vi "Basic_Acquire_Widefield_test.vi"() -> ()   [LabVIEW 2009]
uses:
  <vilib>/vision/Image Controls.llb/IMAQ Image.ctl
  <vilib>/userDefined/High Color/IMAQdx.ctl
  Widefield_globals.vi
  <vilib>/DAQmx/create/channels.llb/DAQmx Create Channel (DO-Digital Output).vi
  <vilib>/DAQmx/configure/timing.llb/DAQmx Timing (Implicit).vi
  <vilib>/DAQmx/create/channels.llb/DAQmx Create Channel (CO-Pulse Generation-Ticks).vi
  <vilib>/Platform/TimedLoop/XDataNode/XDataNode.xnode
  <vilib>/Platform/TimedLoop/XDataNode/loadlvalarms.vi
  <vilib>/Platform/TimedLoop/XDataNode/timing_clust.ctl
  <vilib>/Platform/TimedLoop/XDataNode/nitl_modes.ctl
  <vilib>/Platform/TimedLoop/XDataNode/wakeup.ctl
  <vilib>/DAQmx/write.llb/DAQmx Write (Digital Bool 1Line 1Point).vi
  Program Files/National Instruments/LabVIEW 2009/resource/objmgr/imaqdx.rc
  <vilib>/vision/driver/NI_Vision_Acquisition_Software.lvlib
  <vilib>/Platform/TimedLoop/XDataNode/XDNodeRunTimeDep.lvlib
panel:
  in  "y":dbl
  out "x*y":dbl
  out "RatioIm 2":u8[][](graph)
  out "frame number":i32
  out "IMAQ session":T1 caption="Session Out"
  out "frame times":i32[](array[numeric])
  out "error out":errorcluster
  out "LED settle":i32
  out "Control LED?":bool
  out "stim tag":string
  out "SF file":string
  out "One Bulb?":bool
  out "File Path":path
  out "SingleFrames":bool
  out "empty frame":dbl[][](array[numeric])
  out "Resolution":u32[](array[numeric])
  out "Experiment Sequence":dbl[][](array[numeric])
  out "settings":sgl[](array[numeric])
  out "Buff Img":T2
  out "COString":string
  in  "Offset (32768 default)":u32=32768
  in  "Contrast (600000 default)":u32=600000
  in  "Pause":bool=TRUE
  out "ExpOrderRefnum":refnum<file>
  out "Subframes":u32
  out "DCSAir":dbl[][](array[numeric])
  out "DCOdor":dbl[][](array[numeric])
  out "DCAir":dbl[][](array[numeric])
  out "TiffRefnum":refnum<file>
  out "Indices":i32[](array[numeric])
  out "Frames SAir":u32
  out "Odors:":u32
  out "StopAcq":bool
  in  "Stop":bool=TRUE
  out "Odor #":i32=50
  out "Repeats:":i32=1
  out "Repeat #":i32=1
  out "Frames Odor":u32
  out "Frames Air":u32
  out "Status":string
  out "Stimulus #":i32
  in  "start":bool=TRUE
  # "Filtered Ratio Image"
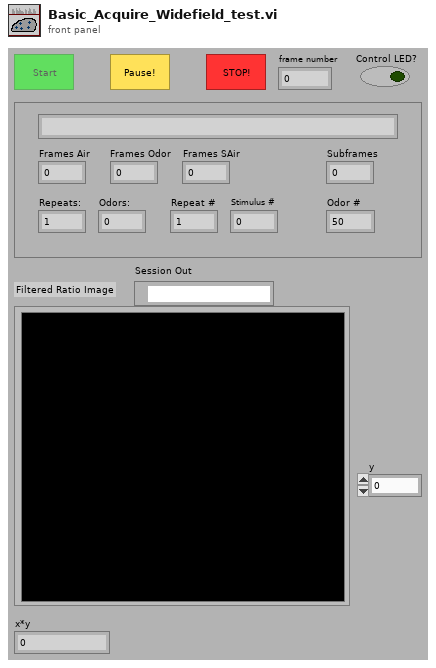
[diagram p1: front panel]
types:
  T1 = typedef "IMAQdx.ctl" = refnum<k21>
  T2 = typedef "IMAQ Image.ctl" = refnum<image>
  T3 = enum16{"open", "replace", "create", "open or create", "replace or create", "replace or create with confirmation"}
  T4 = typedef "XDNodeRunTimeDep.lvlib/timing_clust.ctl" = cluster{"Expected End [f-1]":u64, "Actual End [f-1]":u64, "Finished Late? [f-1]":bool, "Expected End [i-1]":u64, "Actual End [i-1]":u64, "Finished Late? [i-1]":bool, "Expected Start [i]":u64, "Actual Start [i]":u64, "Expected Start [f]":u64, "Actual Start [f]":u64, "Source Name":string, "Structure Name":string, "Period":i64, "Deadline":i64, "Offset":i64, "Start":i64, "Priority":i32, "Timeout":i32, "Mode":T5, "Wakeup Reason":T6, "Error":errorcluster, "Source Type":string, "Secondary Source Type":string, "Global End Time":u64, "Global Start Time":u64, "Frame Duration":u64, "Iteration Duration":u64, "Assigned CPU":i32, "I/O Scan Engine Mode":u32}
  T5 = typedef "XDNodeRunTimeDep.lvlib/nitl_modes.ctl" = enum32{"No Change", "Process missed periods, maintain original phase", "Discard missed periods, maintain original phase", "Process missed periods, ignore original phase", "Discard missed periods, ignore original phase"}
  T6 = typedef "XDNodeRunTimeDep.lvlib/wakeup.ctl" = enum32{"Normal", "Aborted", "Asynchronous wakeup", "Timing source error", "Timed loop error", "Timeout"}
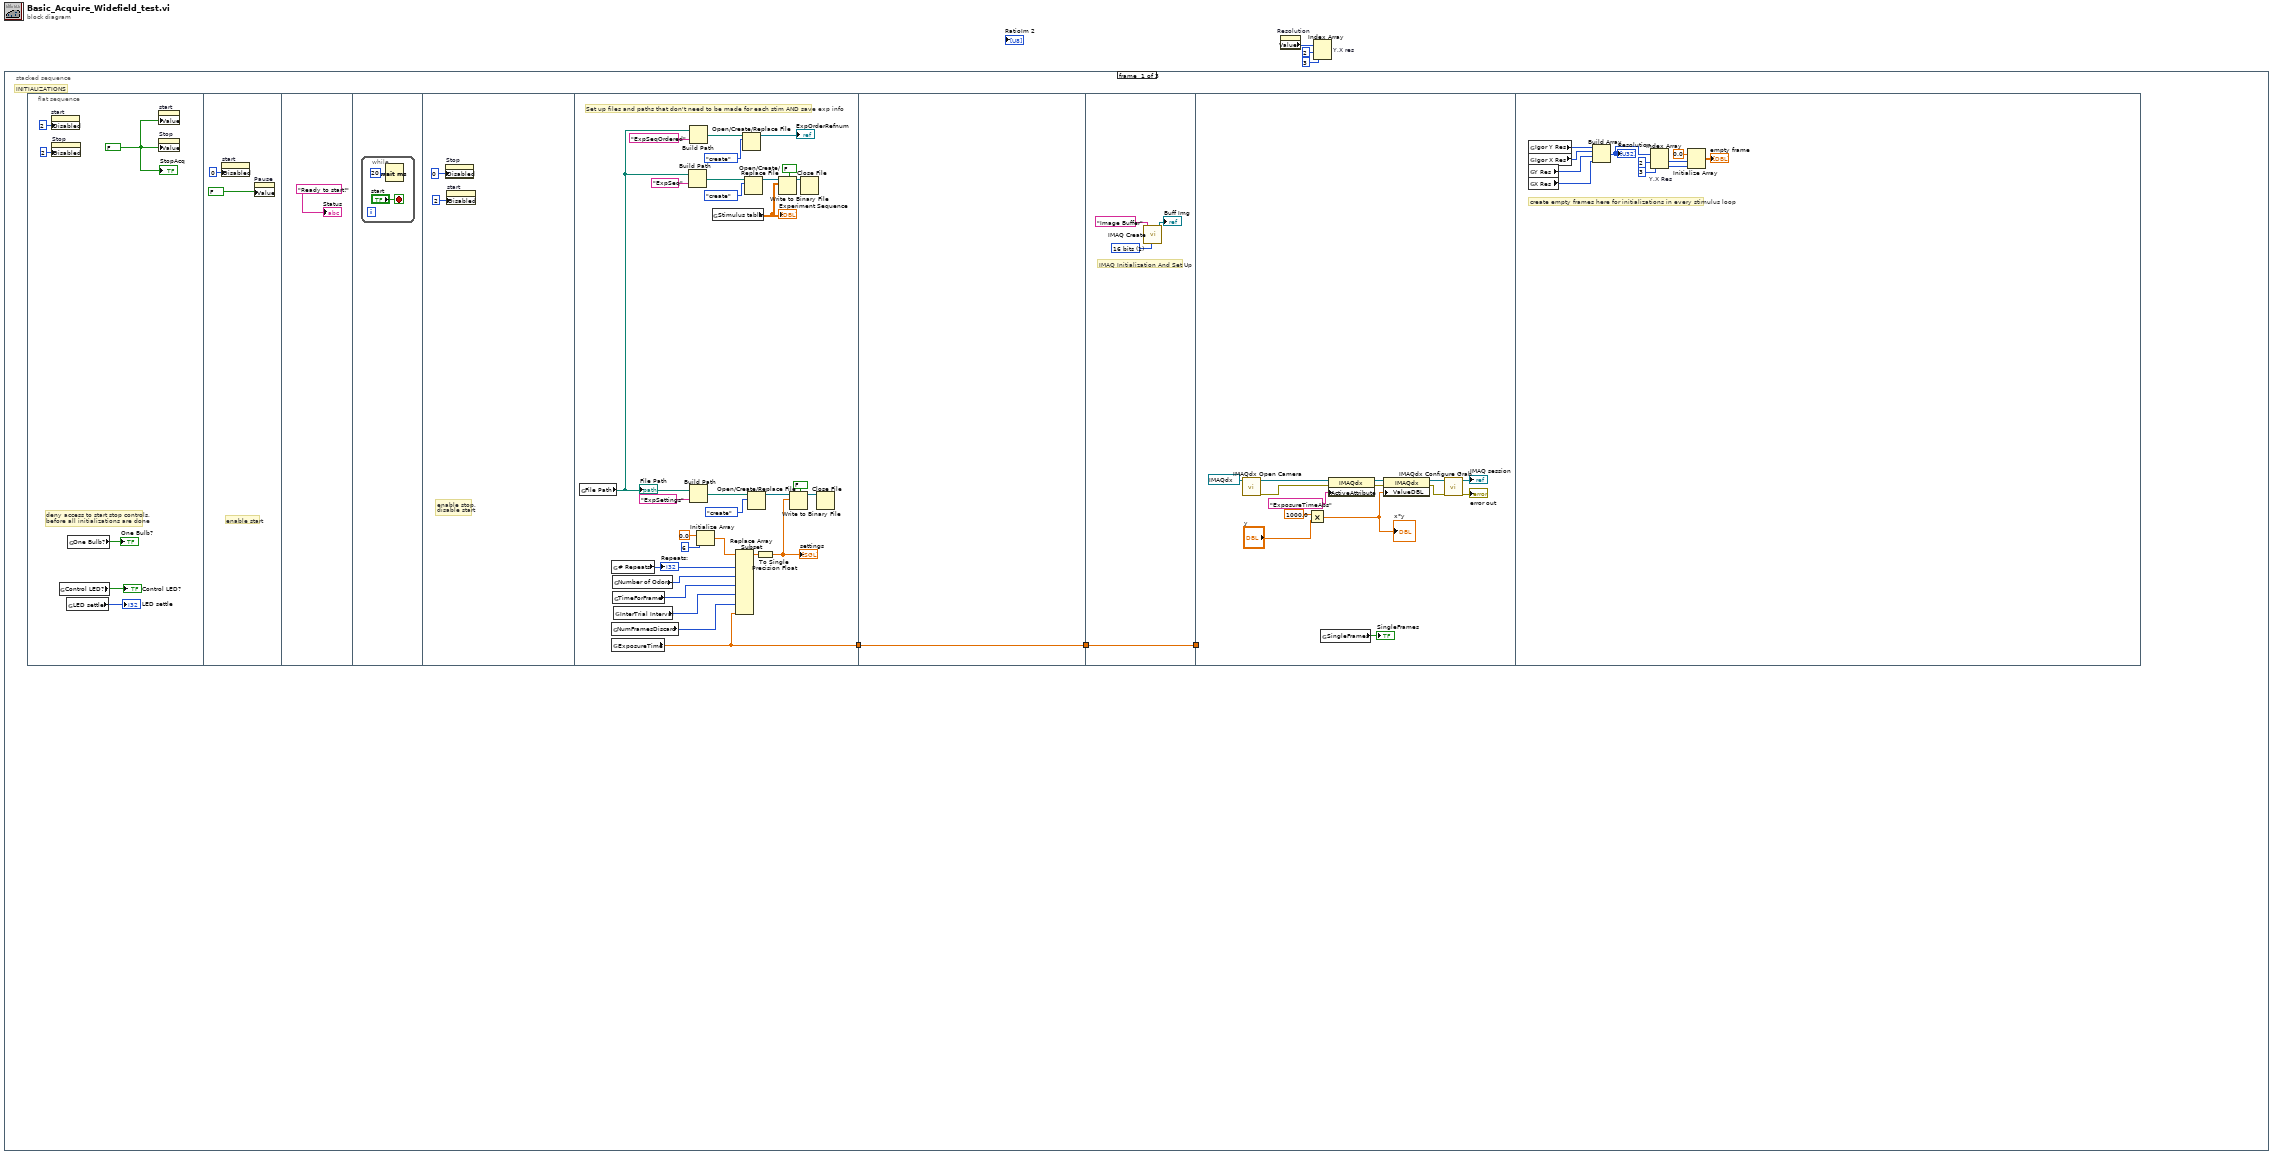
[diagram p0: block diagram]
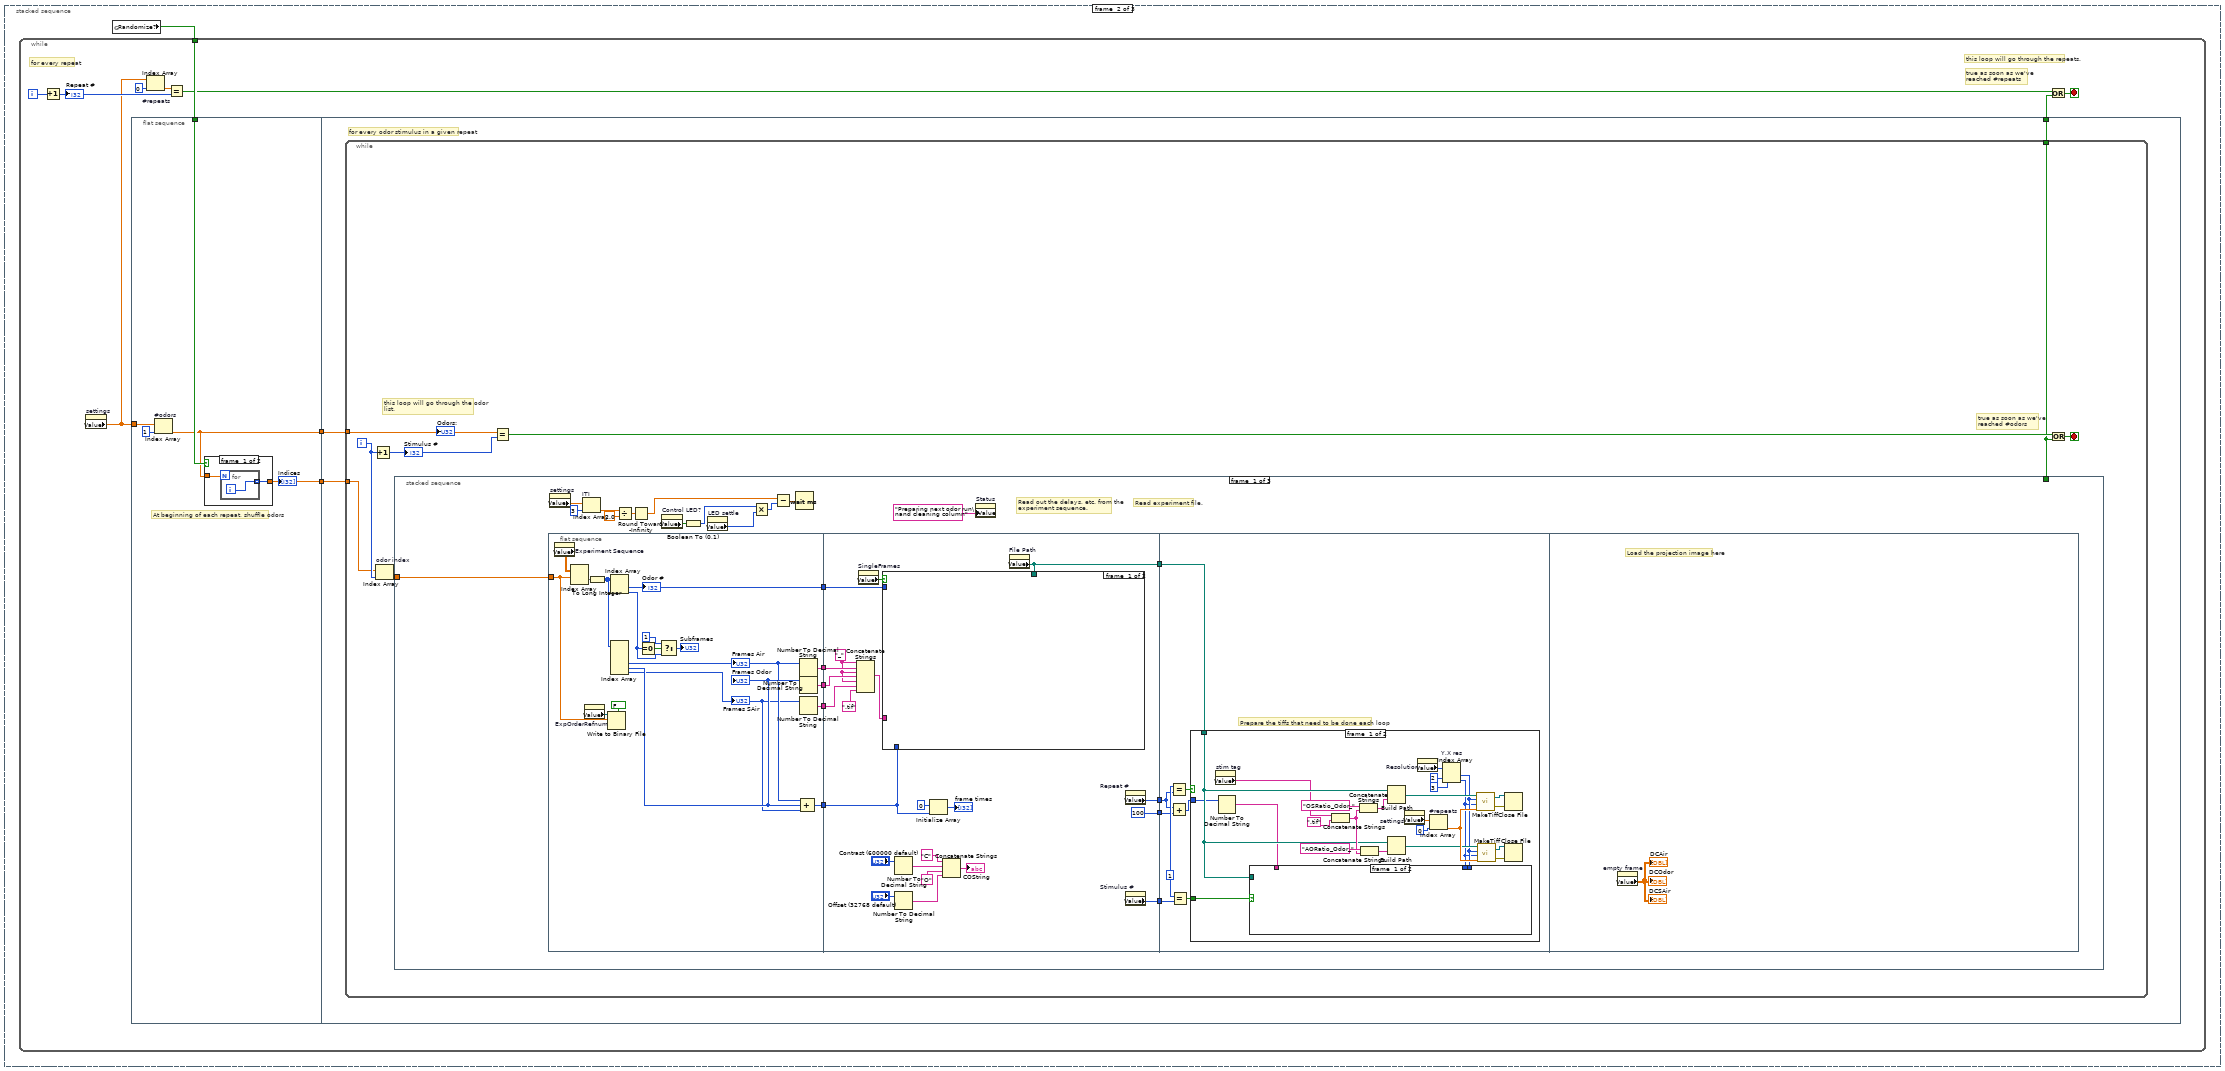
[diagram p2: hidden frame]
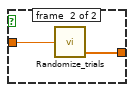
[diagram p3: hidden frame]
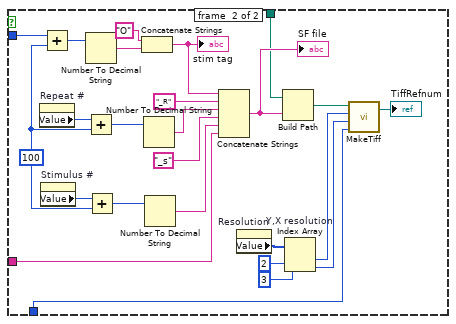
[diagram p4: hidden frame]
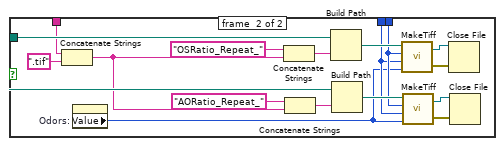
[diagram p5: hidden frame]
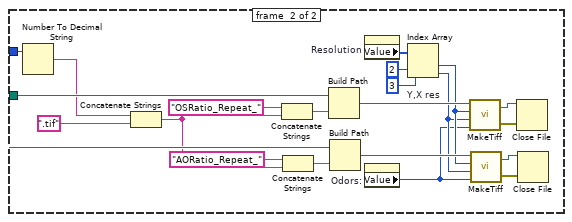
[diagram p7: hidden frame]
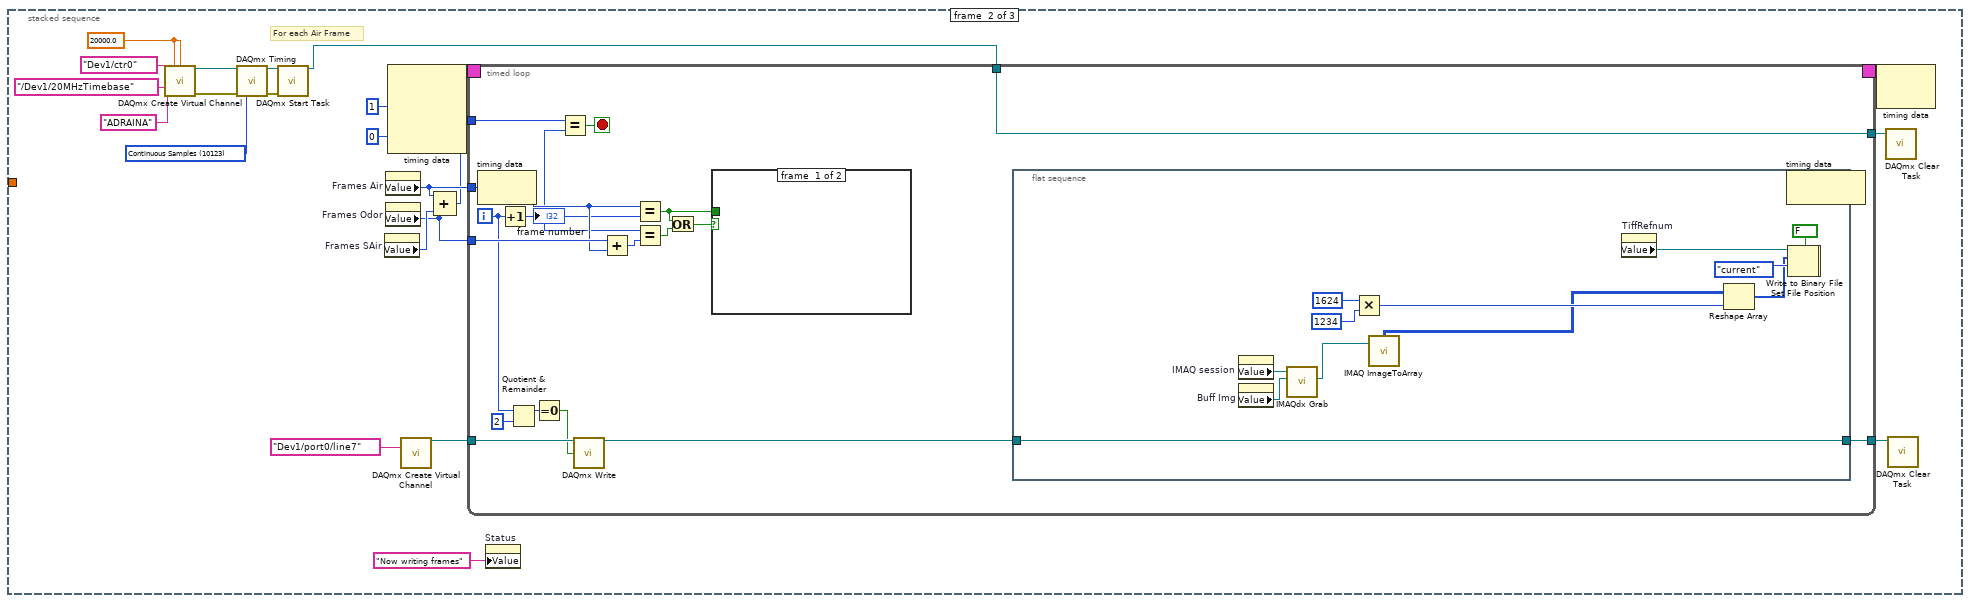
[diagram p8: hidden frame]
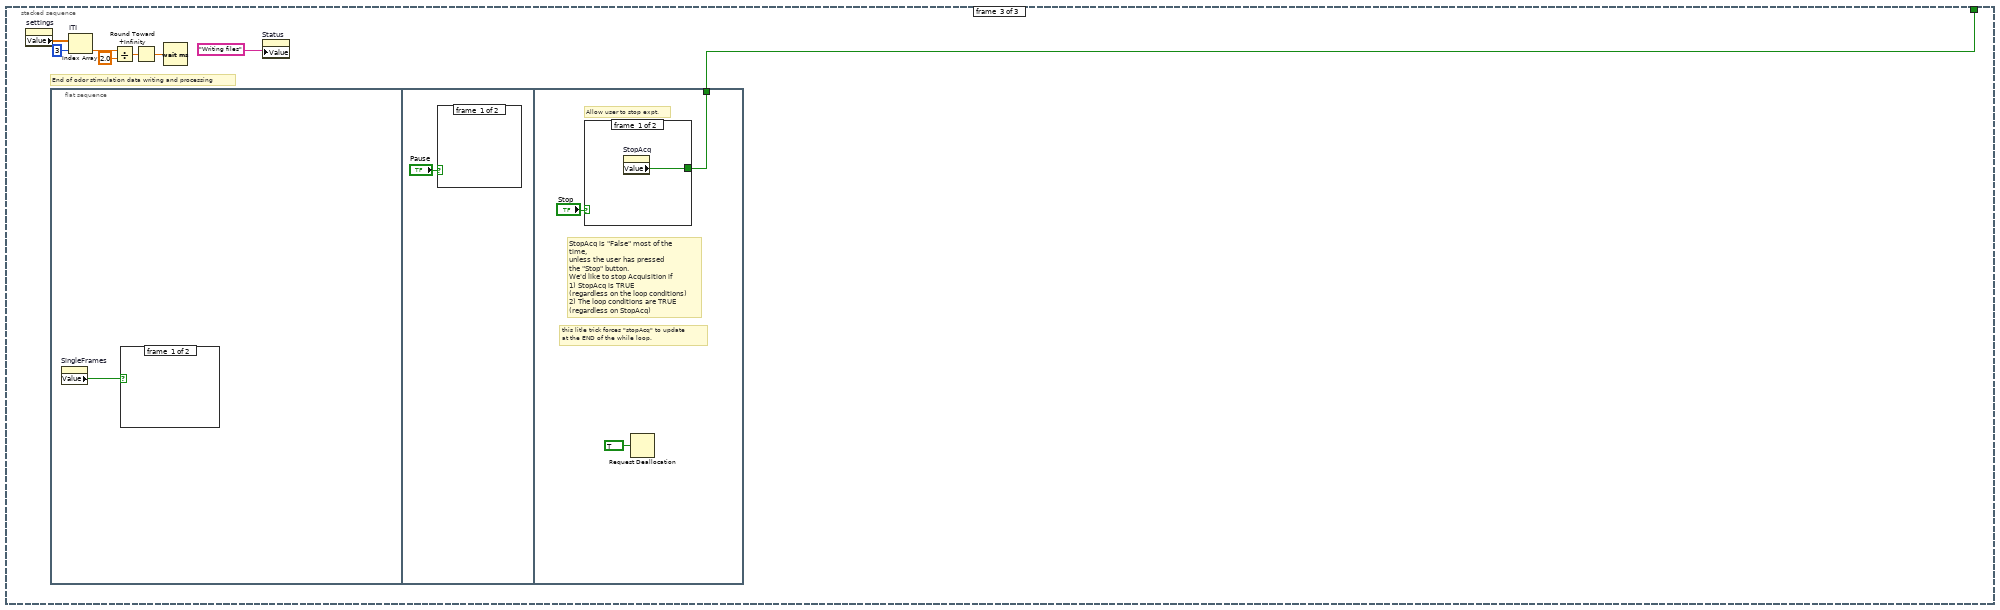
[diagram p11: hidden frame]
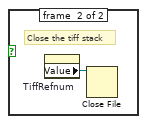
[diagram p12: hidden frame]
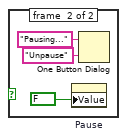
[diagram p13: hidden frame]
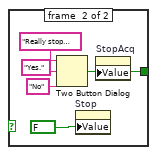
[diagram p14: hidden frame]
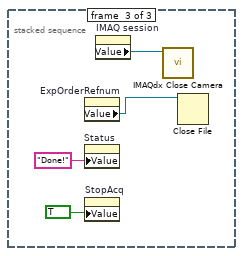
[diagram p15: hidden frame]
diagram:
  n1 = stacked-sequence {
    frame #0 {
      # "INITIALIZATIONS"
      n2 = flat-sequence {
        tunnel: [w21] -> w4
        tunnel: [w49] -> w5
        tunnel: w4 -> [w49]
        tunnel: [w50] -> w6
        tunnel: w5 -> [w50]
        tunnel: w6 -> [_]
        frame #0 {
          w10 = FALSE ("Stop")
          # "deny access to start stop controls, \nbefore all initializations are done"
          n3 = property on="start" class="Boolean (strict)"("Disabled"=u8 2) -> ()  [unwired: 2 in, 2 out]
          n4 = property on="Stop" class="Bool (strict)"("Disabled"=u8 2) -> ()  [unwired: 2 in, 2 out]
          n5 = global read "Widefield_globals.vi" "Control LED?"() -> (→"Control LED?":bool)
          n6 = global read "Widefield_globals.vi" "LED settle"() -> (→"LED settle":i32)
          n7 = global read "Widefield_globals.vi" "One Bulb?"() -> (→"One Bulb?":bool)
          n8 = property on="start" class="Boolean (strict)"("Value"=w10) -> ()  [unwired: 2 in, 2 out]
          n9 = property on="Stop" class="Bool (strict)"("Value"=w10) -> ()  [unwired: 2 in, 2 out]
          "StopAcq" <- w10
        }
        frame #1 {
          # "enable start"
          n10 = property on="start" class="Boolean (strict)"("Disabled"=u8 0) -> ()  [unwired: 2 in, 2 out]
          n11 = property on="Pause" class="Bool (strict)"("Value"=FALSE ("Pause")) -> ()  [unwired: 2 in, 2 out]
        }
        frame #2 {
          "Status" <- "Ready to start!" ("Status")
        }
        frame #3 {
          n12 = while {
            stop <- "start" stop-if-true
            n13 = Wait (ms)(milliseconds to wait=u32 20) -> ()  [unwired: 1 out]
          }
        }
        frame #4 {
          # "enable stop,\ndisable start"
          n14 = property on="Stop" class="Bool (strict)"("Disabled"=u8 0) -> ()  [unwired: 2 in, 2 out]
          n15 = property on="start" class="Boolean (strict)"("Disabled"=u8 2) -> ()  [unwired: 2 in, 2 out]
        }
        frame #5 {
          # "Set up files and paths that don't need to be made for each stim AND save exp info"
          n16 = global read "Widefield_globals.vi" "File Path"() -> (w27:path)
          "File Path" <- w27
          n17 = global read "Widefield_globals.vi" "NumFramesDiscard"() -> (w22:i32)
          n18 = global read "Widefield_globals.vi" "# Repeats"() -> (w25:u16)
          "Repeats:" <- w25
          n19 = global read "Widefield_globals.vi" "ExposureTime"() -> (w21:dbl)
          n20 = global read "Widefield_globals.vi" "Number of Odors"() -> (w24:u32)
          n21 = global read "Widefield_globals.vi" "TimeForFrame"() -> (w20:u32)
          n22 = global read "Widefield_globals.vi" "InterTrial Interval"() -> (w23:i32)
          n23 = Build Path(base path=w27, name or relative path="ExpSeq" ("string")) -> (appended path=w40:path)
          n24 = Build Path(base path=w27, name or relative path="ExpSeqOrdered" ("string")) -> (appended path=w30:path)
          n25 = Build Path(base path=w27, name or relative path="ExpSettings" ("string")) -> (appended path=w38:path)
          n26 = Initialize Array(sgl 0.0 ("element"), 6 ("dimension size")) -> (w34:sgl[])
          n27 = global read "Widefield_globals.vi" "Stimulus table"() -> (w26:dbl[][])
          "Experiment Sequence" <- w26
          n28 = Replace Array Subset(array=w34, new element #1=w25, new element #2=w24, new element #3=w20, new element #4=w23, new element #5=w22, new element #6=w21) -> (w33:sgl[])  [unwired: 6 in]
          n29 = Open/Create/Replace File(file path (use dialog)=w30, operation (0:open)=T3."create") -> (refnum out=→"ExpOrderRefnum":refnum<file>)  [unwired: 1 in, 5 out]
          n30 = Open/Create/Replace File(file path (use dialog)=w40, operation (0:open)=T3."create") -> (refnum out=w47:refnum<file>)  [unwired: 1 in, 5 out]
          n31 = Open/Create/Replace File(file path (use dialog)=w38, operation (0:open)=T3."create") -> (refnum out=w46:refnum<file>)  [unwired: 1 in, 5 out]
          n32 = To Single Precision Float(number=w33) -> (single precision float=w32:sgl[])
          "settings" <- w32
          n33 = Write to Binary File(file (use dialog)=w47, data=w26, 5:FALSE ("prepend array or string size? (T)")) -> (refnum out=w48:refnum<file>)  [unwired: 1 in, 4 out]
          n34 = Write to Binary File(file (use dialog)=w46, data=w32, 5:FALSE ("prepend array or string size? (T)")) -> (refnum out=w31:refnum<file>)  [unwired: 1 in, 4 out]
          n35 = Close File(refnum=w48) -> ()  [unwired: 1 in, 2 out]
          n36 = Close File(refnum=w31) -> ()  [unwired: 1 in, 2 out]
        }
        frame #6 {
        }
        frame #7 {
          w53 = u32 1 items=["8 bits", "16 bits", "Float", "Complex", "RGB", "HSL"] ("Image Type")
          # "IMAQ Initialization And Set Up"
          n37 = call "IMAQ Create"("Image Name"="Image Buffer", "Image Type"=w53) -> ("New Image"=→"Buff Img":T2)  [unwired: 2 in, 2 out]
        }
        frame #8 {
          n38 = call <vilib>:"IMAQdx Open Camera.vi"("Session In"=T1 "cam0") -> ("error out"=w63:errorcluster, "Session Out"=w62:T1)  [unwired: 2 in, 7 out]
          n39 = Multiply(x=1000.0 ("y"), y="y") -> (x*y=w57:dbl)
          "x*y" <- w57
          n40 = global read "Widefield_globals.vi" "SingleFrames"() -> (→"SingleFrames":bool)
          n41 = property class="IMAQdx"(reference=w62, error in=w63, "ActiveAttribute"="ExposureTimeAbs" ("Camera Attribute")) -> (reference out=w58:T1, error out=w59:errorcluster)
          n42 = property class="IMAQdx"(reference=w58, error in=w59, "ValueDBL"=w57) -> (reference out=w65:T1, error out=w61:errorcluster)
          n43 = call <vilib>:"IMAQdx Configure Grab.vi"("error in"=w61, "Session In"=w65) -> ("error out"=→"error out":errorcluster, "Session Out"=→"IMAQ session":T1)  [unwired: 8 out]
        }
        frame #9 {
          # "create empty frames here for initializations in every stimulus loop"
          n44 = global read "Widefield_globals.vi" "Y Res"() -> (w69:u32)
          n45 = global read "Widefield_globals.vi" "X Res"() -> (w68:u32)
          n46 = global read "Widefield_globals.vi" "Igor Y Res"() -> (w72:u32)
          n47 = global read "Widefield_globals.vi" "Igor X Res"() -> (w71:u32)
          n48 = Build Array(w72, w71, w69, w68) -> (w70:u32[])
          "Resolution" <- w70
          n49 = Index Array "Y,X Res"(array=w70, index #1=2 ("index"), index #2=3 ("index")) -> (element #1=w78:u32, element #2=w77:u32)
          n50 = Initialize Array(0.0 ("element"), w78, w77) -> (→"empty frame":dbl[][])
        }
      }
    }
    frame #1 {
      n51 = global read "Widefield_globals.vi" "Randomize?"() -> (w79:bool)
      n52 = while {
        tunnel: w79 -> [w88]
        i -> [w83]
        stop <- w90 stop-if-true
        # "for every repeat"
        # "this loop will go through the repeats."
        # "true as soon as we've\nreached #repeats"
        n53 = Increment(x=w83) -> (x+1=w89:i32)
        "Repeat #" <- w89
        n54 = property on="settings" class="Arr (strict)"() -> ("Value"=w85:sgl[])  [unwired: 2 in, 2 out]
        n55 = flat-sequence {
          tunnel: w85 -> [w95]
          tunnel: w88 -> [w93]
          tunnel: [w92] -> w87
          tunnel: [w91] -> w86
          tunnel: w87 -> [w103]
          tunnel: w86 -> [w102]
          tunnel: [w101] -> w81
          frame #0 {
            # "At beginning of each repeat, shuffle odors"
            n56 = Index Array "#odors"(array=w95, index=1) -> (element=w92:sgl)
            n57 = case shown="True" w93 {
              tunnel: [w96 w100] -> w91
              tunnel: w92 -> [w97 w99]
              frame #0 {
                n58 = for {
                  N: w97 -> [_]
                  tunnel: [w98] -> w96 mode=indexing
                  i -> [w98]
                }
              }
              frame #1 {
                n59 = call "Randomize_trials.vi"("ArraySize"=w99) -> ("Randomized"=w100:dbl[])  [unwired: 2 in]
              }
            }
            "Indices" <- w91
          }
          frame #1 {
            # "for every odor stimulus in a given repeat"
            n60 = while {
              tunnel: w103 -> [w110]
              tunnel: w102 -> [w107]
              tunnel: [w105] -> w101
              i -> [w109]
              stop <- w111 stop-if-true
              # "this loop will go through the odor\nlist."
              # "true as soon as we've\nreached #odors"
              n61 = Increment(x=w109) -> (x+1=w104:i32)
              "Stimulus #" <- w104
              n62 = Index Array "odor index"(array=w107, index=w109) -> (element=w108:dbl)
              n63 = stacked-sequence {
                tunnel: w108 -> [w133 _ _]
                tunnel: [_ _ w343] -> w105
                frame #0 {
                  # "Read experiment file."
                  # "Read out the delays, etc. from the\nexperiment sequence."
                  n64 = flat-sequence {
                    tunnel: [w149] -> w132
                    tunnel: [w148] -> w131
                    tunnel: [w147] -> w130
                    tunnel: [w146] -> w129
                    tunnel: [w145] -> w128
                    tunnel: w133 -> [w137]
                    tunnel: [w165] -> w127
                    tunnel: [w166] -> w126
                    tunnel: [w164] -> w125
                    tunnel: w128 -> [w154]
                    tunnel: w129 -> [w160]
                    tunnel: w130 -> [w161]
                    tunnel: w131 -> [w162]
                    tunnel: w132 -> [w163]
                    tunnel: [100 ("y")] -> w117
                    tunnel: w127 -> [w200]
                    tunnel: w126 -> [w205]
                    tunnel: w125 -> [w204]
                    tunnel: w117 -> [w201]
                    frame #0 {
                      n65 = property on="Experiment Sequence" class="Arr (strict)"() -> ("Value"=w144:dbl[][])  [unwired: 2 in, 2 out]
                      n66 = Index Array(array=w144, index (row)=w137) -> (element=w143:dbl[])  [unwired: 1 in]
                      n67 = property on="ExpOrderRefnum" class="Ref (strict)"() -> ("Value"=w150:refnum<file>)  [unwired: 2 in, 2 out]
                      n68 = To Long Integer(number=w143) -> (32bit integer=w139:i32[])
                      n69 = Write to Binary File(file (use dialog)=w150, data=w137, 5:FALSE ("prepend array or string size? (T)")) -> ()  [unwired: 1 in, 5 out]
                      n70 = Index Array(array=w139) -> (element #1=w146:i32, element #2=w136:i32)  [unwired: 2 in]
                      "Odor #" <- w146
                      n71 = Index Array(array=w139) -> (element #3=w135:i32, element #4=w138:i32, element #5=w134:i32)  [unwired: 5 in, 2 out]
                      "Frames Air" <- w135
                      "Frames Odor" <- w138
                      "Frames SAir" <- w134
                      n72 = Equal To 0?(x=w136) -> (x = 0?=w142:bool)
                      n73 = Select(t=1, s=w142, f=w136) -> (s? t:f=→"Subframes":i32)
                      n74 = Number To Decimal String(number=w135) -> (decimal integer string=w149:string)  [unwired: 1 out]
                      n75 = Number To Decimal String(number=w138) -> (decimal integer string=w148:string)  [unwired: 1 out]
                      n76 = Number To Decimal String(number=w134) -> (decimal integer string=w147:string)  [unwired: 1 out]
                      n77 = Compound Arithmetic op=ADD(w135, w138, w134) -> (w145:i32)
                    }
                    frame #1 {
                      w157 = "_" ("string")
                      n78 = Concatenate Strings(w157, w163, w157, w162, w157, w161, ".tif" ("string")) -> (w158:string)
                      n79 = property on="SingleFrames" class="Bool (strict)"() -> ("Value"=w159:bool)  [unwired: 2 in, 2 out]
                      n80 = Number To Decimal String(number="Contrast (600000 default)") -> (decimal integer string=w169:string)  [unwired: 1 out]
                      n81 = Number To Decimal String(number="Offset (32768 default)") -> (decimal integer string=w168:string)  [unwired: 1 out]
                      n82 = Initialize Array(0 ("element"), w154) -> (→"frame times":i32[])
                      n83 = Concatenate Strings("C" ("string"), w169, "O" ("string"), w168) -> (→"COString":string)
                      n84 = property on="File Path" class="Path"() -> ("Value"=w166:path)  [unwired: 2 in, 2 out]
                      n85 = case shown="True" w159 {
                        tunnel: w160 -> [_ w193]
                        tunnel: w166 -> [_ w181]
                        tunnel: w158 -> [_ w174]
                        tunnel: w154 -> [_ w191]
                        frame #0 {
                        }
                        frame #1 {
                          w192 = 100 ("y")
                          n86 = property on="Repeat #" class="DigNum (strict)"() -> ("Value"=w184:i32)  [unwired: 2 in, 2 out]
                          n87 = property on="Stimulus #" class="DigNum (strict)"() -> ("Value"=w177:i32)  [unwired: 2 in, 2 out]
                          n88 = Add(x=w193, y=w192) -> (x+y=w197:i32)
                          n89 = Number To Decimal String(number=w197) -> (decimal integer string=w179:string)  [unwired: 1 out]
                          n90 = Add(x=w184, y=w192) -> (x+y=w198:i32)
                          n91 = Add(x=w177, y=w192) -> (x+y=w194:i32)
                          n92 = Concatenate Strings("O" ("string"), w179) -> (w178:string)
                          "stim tag" <- w178
                          n93 = Number To Decimal String(number=w198) -> (decimal integer string=w196:string)  [unwired: 1 out]
                          n94 = Number To Decimal String(number=w194) -> (decimal integer string=w175:string)  [unwired: 1 out]
                          n95 = Concatenate Strings(w178, "_R" ("string"), w196, "_s" ("string"), w175, w174) -> (w183:string)
                          "SF file" <- w183
                          n96 = property on="Resolution" class="Arr (strict)"() -> ("Value"=w189:u32[])  [unwired: 2 in, 2 out]
                          n97 = Build Path(base path=w181, name or relative path=w183) -> (appended path=w182:path)
                          n98 = Index Array "Y,X resolution"(array=w189, index #1=2 ("index"), index #2=3 ("index")) -> (element #1=w186:u32, element #2=w185:u32)
                          n99 = call "MakeTiff.vi"("z"=w191, "X"=w185, "Y"=w186, "file path"=w182) -> ("refnum tif"=→"TiffRefnum":refnum<file>)  [unwired: 1 out]
                        }
                      }
                      n100 = property on="Repeat #" class="DigNum (strict)"() -> ("Value"=w165:i32)  [unwired: 2 in, 2 out]
                      n101 = property on="Stimulus #" class="DigNum (strict)"() -> ("Value"=w164:i32)  [unwired: 2 in, 2 out]
                    }
                    frame #2 {
                      w203 = 1 ("x")
                      # "Prepare the tiffs that need to be done each loop"
                      n102 = Equal?(x=w203, y=w200) -> (x = y?=w206:bool)
                      n103 = Add(x=w200, y=w201) -> (x+y=w199:i32)
                      n104 = Equal?(x=w203, y=w204) -> (x = y?=w202:bool)
                      n105 = case shown="False" w206 {
                        tunnel: w205 -> [w214 w251]
                        tunnel: w199 -> [w210 w250]
                        tunnel: w202 -> [w209 w249]
                        frame #0 {
                          n106 = property on="stim tag" class="Str"() -> ("Value"=w208:string)  [unwired: 2 in, 2 out]
                          n107 = Number To Decimal String(number=w210) -> (decimal integer string=w211:string)  [unwired: 1 out]
                          n108 = Concatenate Strings(w208, ".tif" ("string")) -> (w223:string)
                          n109 = Concatenate Strings("OSRatio_Odor_" ("string"), w223) -> (w225:string)
                          n110 = Concatenate Strings("AORatio_Odor_" ("string"), w223) -> (w222:string)
                          n111 = Build Path(base path=w214, name or relative path=w222) -> (appended path=w215:path)
                          n112 = Build Path(base path=w214, name or relative path=w225) -> (appended path=w227:path)
                          n113 = property on="settings" class="Arr (strict)"() -> ("Value"=w217:sgl[])  [unwired: 2 in, 2 out]
                          n114 = property on="Resolution" class="Arr (strict)"() -> ("Value"=w221:u32[])  [unwired: 2 in, 2 out]
                          n115 = Index Array "#repeats"(array=w217, index=0) -> (element=w216:sgl)
                          n116 = Index Array "Y,X res"(array=w221, index #1=2 ("index"), index #2=3 ("index")) -> (element #1=w213:u32, element #2=w212:u32)
                          n117 = case shown="True" w209 {
                            tunnel: w214 -> [_ w238]
                            tunnel: w213 -> [_ w237]
                            tunnel: w212 -> [_ w236]
                            tunnel: w211 -> [_ w234]
                            frame #0 {
                            }
                            frame #1 {
                              n118 = Concatenate Strings(w234, ".tif" ("string")) -> (w235:string)
                              n119 = property on="Odors:" class="DigNum (strict)"() -> ("Value"=w233:u32)  [unwired: 2 in, 2 out]
                              n120 = Concatenate Strings("OSRatio_Repeat_" ("string"), w235) -> (w248:string)
                              n121 = Concatenate Strings("AORatio_Repeat_" ("string"), w235) -> (w240:string)
                              n122 = Build Path(base path=w238, name or relative path=w248) -> (appended path=w239:path)
                              n123 = Build Path(base path=w238, name or relative path=w240) -> (appended path=w242:path)
                              n124 = call "MakeTiff.vi"("z"=w233, "X"=w236, "Y"=w237, "file path"=w239) -> ("error out"=w246:errorcluster, "refnum tif"=w245:refnum<file>)
                              n125 = call "MakeTiff.vi"("z"=w233, "X"=w236, "Y"=w237, "file path"=w242) -> ("error out"=w243:errorcluster, "refnum tif"=w244:refnum<file>)
                              n126 = Close File(refnum=w245, error in=w246) -> ()  [unwired: 2 out]
                              n127 = Close File(refnum=w244, error in=w243) -> ()  [unwired: 2 out]
                            }
                          }
                          n128 = call "MakeTiff.vi"("z"=w216, "X"=w212, "Y"=w213, "file path"=w227) -> ("error out"=w228:errorcluster, "refnum tif"=w229:refnum<file>)
                          n129 = call "MakeTiff.vi"("z"=w216, "X"=w212, "Y"=w213, "file path"=w215) -> ("error out"=w230:errorcluster, "refnum tif"=w231:refnum<file>)
                          n130 = Close File(refnum=w229, error in=w228) -> ()  [unwired: 2 out]
                          n131 = Close File(refnum=w231, error in=w230) -> ()  [unwired: 2 out]
                        }
                        frame #1 {
                          n132 = case shown="True" w249 {
                            tunnel: w251 -> [_ w259]
                            tunnel: w250 -> [_ w254]
                            frame #0 {
                            }
                            frame #1 {
                              n133 = Number To Decimal String(number=w254) -> (decimal integer string=w255:string)  [unwired: 1 out]
                              n134 = Concatenate Strings(w255, ".tif" ("string")) -> (w256:string)
                              n135 = Concatenate Strings("OSRatio_Repeat_" ("string"), w256) -> (w269:string)
                              n136 = Concatenate Strings("AORatio_Repeat_" ("string"), w256) -> (w261:string)
                              n137 = Build Path(base path=w259, name or relative path=w269) -> (appended path=w260:path)
                              n138 = Build Path(base path=w259, name or relative path=w261) -> (appended path=w263:path)
                              n139 = property on="Resolution" class="Arr (strict)"() -> ("Value"=w272:u32[])  [unwired: 2 in, 2 out]
                              n140 = property on="Odors:" class="DigNum (strict)"() -> ("Value"=w253:u32)  [unwired: 2 in, 2 out]
                              n141 = Index Array "Y,X res"(array=w272, index #1=2 ("index"), index #2=3 ("index")) -> (element #1=w258:u32, element #2=w257:u32)
                              n142 = call "MakeTiff.vi"("z"=w253, "X"=w257, "Y"=w258, "file path"=w260) -> ("error out"=w267:errorcluster, "refnum tif"=w266:refnum<file>)
                              n143 = call "MakeTiff.vi"("z"=w253, "X"=w257, "Y"=w258, "file path"=w263) -> ("error out"=w264:errorcluster, "refnum tif"=w265:refnum<file>)
                              n144 = Close File(refnum=w266, error in=w267) -> ()  [unwired: 2 out]
                              n145 = Close File(refnum=w265, error in=w264) -> ()  [unwired: 2 out]
                            }
                          }
                        }
                      }
                    }
                    frame #3 {
                      # "Load the projection image here"
                      n146 = property on="empty frame" class="Arr (strict)"() -> ("Value"=→"DCAir" →"DCOdor" →"DCSAir":dbl[][])  [unwired: 2 in, 2 out]
                    }
                  }
                  n147 = property on="settings" class="Arr (strict)"() -> ("Value"=w124:sgl[])  [unwired: 2 in, 2 out]
                  n148 = Index Array "ITI"(array=w124, index=3) -> (element=w122:sgl)
                  n149 = Divide(x=w122, y=sgl 2.0) -> (x/y=w120:sgl)
                  n150 = Round Toward -Infinity(1:w120) -> (0:w119:sgl)
                  n151 = property on="Control LED?" class="Bool (strict)"() -> ("Value"=w115:bool)  [unwired: 2 in, 2 out]
                  n152 = Boolean To (0,1)(Boolean=w115) -> (0, 1=w113:i16)
                  n153 = property on="LED settle" class="DigNum (strict)"() -> ("Value"=w112:i32)  [unwired: 2 in, 2 out]
                  n154 = Multiply(x=w113, y=w112) -> (x*y=w114:i32)
                  n155 = Subtract(x=w119, y=w114) -> (x-y=w116:sgl)
                  n156 = Wait (ms)(milliseconds to wait=w116) -> ()  [unwired: 1 out]
                  n157 = property on="Status" class="Str"("Value"="Preparing next odor run\nand cleaning column" ("Status")) -> ()  [unwired: 2 in, 2 out]
                }
                frame #1 {
                  w284 = 10123 items=["Finite Samples"=10178, "Continuous Samples"=10123, "Hardware Timed Single Point"=12522] ("sample mode")
                  w278 = 20000.0 ("duty cycle")
                  # "For each Air Frame"
                  n158 = call-poly <vilib>:"DAQmx Create Virtual Channel.vi"("high ticks"=w278, "low ticks"=w278, "counter"=tag "Dev1/ctr0", "name to assign"="ADRAINA", "source of ticks"=tag "/Dev1/20MHzTimebase") -> ("task out"=w286:refnum<k21>, "error out"=w285:errorcluster)  [unwired: 9 in]
                  n159 = call-poly <vilib>:"DAQmx Timing.vi"("task/channels in"=w286, "sample mode"=w284, "error in"=w285) -> ("task out"=w283:refnum<k21>, "error out"=w282:errorcluster)  [unwired: 11 in]
                  n160 = call <vilib>:"DAQmx Start Task.vi"("task/channels in"=w283, "error in"=w282) -> ("task out"=w281:refnum<k21>)  [unwired: 12 in, 1 out]
                  n161 = property on="Frames SAir" class="DigNum (strict)"() -> ("Value"=w295:u32)  [unwired: 2 in, 2 out]
                  n162 = property on="Frames Air" class="DigNum (strict)"() -> ("Value"=w294:u32)  [unwired: 2 in, 2 out]
                  n163 = property on="Frames Odor" class="DigNum (strict)"() -> ("Value"=w293:u32)  [unwired: 2 in, 2 out]
                  n164 = node-c288(i64 1 ("Period"), 0 ("Processor")) -> (w289:T4)  [unwired: 2 in]
                  n165 = call-poly <vilib>:"DAQmx Create Virtual Channel.vi"("lines"=tag "Dev1/port0/line7") -> ("task out"=w291:refnum<k21>)  [unwired: 13 in, 1 out]
                  n166 = Compound Arithmetic op=ADD(w294, w293, w295) -> (w287:u32)
                  n167 = timed-loop {
                    tunnel: w294 -> [w311]
                    tunnel: w293 -> [w313]
                    tunnel: w291 -> [w304]
                    tunnel: [w301] -> w290
                    timing: w289 -> [_]
                    timing-out: [_] -> w288
                    tunnel: w287 -> [w298]
                    tunnel: w281 -> [w297]
                    tunnel: [w297] -> w280
                    i -> [w307]
                    stop <- w300 stop-if-true
                    n168 = node-c288() -> ()  [unwired: 1 in, 1 out]
                    n169 = Increment(x=w307) -> (x+1=w299:i32)
                    "frame number" <- w299
                    n170 = Quotient & Remainder(x=w307, y=2) -> (x-y*floor(x/y)=w305:i32)  [unwired: 1 out]
                    n171 = Equal To 0?(x=w305) -> (x = 0?=w303:bool)
                    n172 = Equal?(x=w298, y=w299) -> (x = y?=w300:bool)
                    n173 = call-poly <vilib>:"DAQmx Write.vi"("task/channels in"=w304, "data"=w303) -> ("task out"=w302:refnum<k21>)  [unwired: 11 in, 2 out]
                    n174 = Add(x=w313, y=w311) -> (x+y=w312:u32)
                    n175 = Equal?(x=w311, y=w299) -> (x = y?=w308:bool)
                    n176 = Equal?(x=w299, y=w312) -> (x = y?=w309:bool)
                    n177 = Or(x=w308, y=w309) -> (x .or. y?=w310:bool)
                    n178 = case shown="True" w310 {
                      tunnel: w308 -> [_ w330]
                      frame #0 {
                      }
                      frame #1 {
                        n179 = case shown="True" w330 {
                          frame #0 {
                          }
                          frame #1 {
                          }
                        }
                      }
                    }
                    n180 = flat-sequence {
                      tunnel: [w327] -> w301
                      tunnel: w302 -> [w327]
                      frame #0 {
                        n181 = property on="IMAQ session" class="IMAQdx (strict)"() -> ("Value"=w319:refnum<k21>)  [unwired: 2 in, 2 out]
                        n182 = property on="Buff Img" class="IMAQImage (strict)"() -> ("Value"=w320:refnum<image>)  [unwired: 2 in, 2 out]
                        n183 = call <vilib>:"IMAQdx Grab.vi"("Image In"=w320, "Session In"=w319) -> ("Image Out"=w318:T2)  [unwired: 2 in, 7 out]
                        n184 = Multiply(x=u32 1624, y=u32 1234 ("x")) -> (x*y=w329:u32)
                        n185 = call "IMAQ ImageToArray"("Image"=w318) -> ("Image Pixels (U8)"=w321:u8[][])  [unwired: 2 in, 5 out]
                        n186 = property on="TiffRefnum" class="Ref (strict)"() -> ("Value"=w328:refnum<file>)  [unwired: 2 in, 2 out]
                        n187 = Reshape Array(w321, w329) -> (w325:u8[])
                        n188 = Set File Position(refnum=w328, from (0:start)=enum16{"start", "end", "current"}."current" ("pos mode (0:2)")) -> (refnum out=w324:refnum<file>, error out=w323:errorcluster)  [unwired: 1 in, 1 out]
                        n189 = Write to Binary File(file (use dialog)=w324, data=w325, error in=w323, 5:FALSE ("prepend array or string size? (T)")) -> ()  [unwired: 5 out]
                      }
                    }
                    n190 = node-c288() -> ()  [unwired: 1 in, 1 out]
                  }
                  n191 = property on="Status" class="Str"("Value"="Now writing frames" ("String")) -> ()  [unwired: 2 in, 2 out]
                  n192 = node-c288(w288) -> ()  [unwired: 1 out]
                  n193 = call <vilib>:"DAQmx Clear Task.vi"("task in"=w280) -> ()  [unwired: 14 in, 1 out]
                  n194 = call <vilib>:"DAQmx Clear Task.vi"("task in"=w290) -> ()  [unwired: 14 in, 1 out]
                }
                frame #2 {
                  # "End of odor stimulation data writing and processing"
                  n195 = property on="settings" class="Arr (strict)"() -> ("Value"=w342:sgl[])  [unwired: 2 in, 2 out]
                  n196 = flat-sequence {
                    tunnel: [w351] -> w343
                    frame #0 {
                      n197 = property on="SingleFrames" class="Bool (strict)"() -> ("Value"=w344:bool)  [unwired: 2 in, 2 out]
                      n198 = case shown="True" w344 {
                        frame #0 {
                        }
                        frame #1 {
                          # "Close the tiff stack"
                          n199 = property on="TiffRefnum" class="Ref (strict)"() -> ("Value"=w345:refnum<file>)  [unwired: 2 in, 2 out]
                          n200 = Close File(refnum=w345) -> ()  [unwired: 1 in, 2 out]
                        }
                      }
                    }
                    frame #1 {
                      n201 = case shown="True" "Pause" {
                        frame #0 {
                        }
                        frame #1 {
                          n202 = property on="Pause" class="Bool (strict)"("Value"=FALSE ("Pause")) -> ()  [unwired: 2 in, 2 out]
                          n203 = One Button Dialog(message="Pausing...", button name ("OK")="Unpause") -> ()  [unwired: 1 out]
                        }
                      }
                    }
                    frame #2 {
                      # "this litle trick forces \"stopAcq\" to update\nat the END of the while loop."
                      # "StopAcq is \"False\" most of the time, \nunless the user has pressed\nthe \"Stop\" button.\nWe'd like to stop Acquisition if\n1) StopAcq is TRUE \n(regardless on the loop conditions)\n2) The loop conditions are TRUE \n(regardless on StopAcq)"
                      # "Allow user to stop expt."
                      n204 = case shown="True" "Stop" {
                        tunnel: [w353 w354] -> w351
                        frame #0 {
                          n205 = property on="StopAcq" class="Bool (strict)"() -> ("Value"=w353:bool)  [unwired: 2 in, 2 out]
                        }
                        frame #1 {
                          n206 = Two Button Dialog(message="Really stop acquisition after this stimulus?", 1:"No" ("F button name (\"Cancel\")"), 2:"Yes." ("T button name (\"OK\")")) -> (T button?=w354:bool)
                          n207 = property on="Stop" class="Bool (strict)"("Value"=FALSE ("Stop")) -> ()  [unwired: 2 in, 2 out]
                          n208 = property on="StopAcq" class="Bool (strict)"("Value"=w354) -> ()  [unwired: 2 in, 2 out]
                        }
                      }
                      n209 = Request Deallocation(TRUE ("flag")) -> ()
                    }
                  }
                  n210 = Index Array "ITI"(array=w342, index=3) -> (element=w340:sgl)
                  n211 = Divide(x=w340, y=sgl 2.0) -> (x/y=w338:sgl)
                  n212 = Round Toward +Infinity(x=w338) -> (ceil(x): smallest int >= x=w337:sgl)
                  n213 = Wait (ms)(milliseconds to wait=w337) -> ()  [unwired: 1 out]
                  n214 = property on="Status" class="Str"("Value"="Writing files" ("String")) -> ()  [unwired: 2 in, 2 out]
                }
              }
              n215 = Equal?(x=w110, y=w104) -> (x = y?=w106:bool)
              n216 = Or(x=w106, y=w105) -> (x .or. y?=w111:bool)
              "Odors:" <- w110
            }
          }
        }
        n217 = Index Array "#repeats"(array=w85, index=0) -> (element=w84:sgl)
        n218 = Equal?(x=w84, y=w89) -> (x = y?=w82:bool)
        n219 = Or(x=w82, y=w81) -> (x .or. y?=w90:bool)
      }
    }
    frame #2 {
      n220 = property on="ExpOrderRefnum" class="Ref (strict)"() -> ("Value"=w361:refnum<file>)  [unwired: 2 in, 2 out]
      n221 = property on="Status" class="Str"("Value"="Done!" ("Status")) -> ()  [unwired: 2 in, 2 out]
      n222 = property on="StopAcq" class="Bool (strict)"("Value"=TRUE ("StopAcq")) -> ()  [unwired: 2 in, 2 out]
      n223 = property on="IMAQ session" class="IMAQdx (strict)"() -> ("Value"=w359:refnum<k21>)  [unwired: 2 in, 2 out]
      n224 = call <vilib>:"IMAQdx Close Camera.vi"("Session In"=w359) -> ()  [unwired: 1 in, 10 out]
      n225 = Close File(refnum=w361) -> ()  [unwired: 1 in, 2 out]
    }
  }
  n226 = property on="Resolution" class="Arr (strict)"() -> ("Value"=w1:u32[])  [unwired: 2 in, 2 out]
  n227 = Index Array "Y,X res"(array=w1, index #1=2 ("index"), index #2=3 ("index")) -> ()  [unwired: 2 out]
